vi "04Foot_DAQRead.vi"(0 "task/channels in":refnum<k21>, 7 "number of samples per channel":i32=-1, 9 "timeout":dbl=10.0 format="%0.2f", 11 "error in":errorcluster) -> (4 "task out":refnum<k21>, 6 "data":u8[](array[numeric]), 15 "error out":errorcluster)   [LabVIEW 2015]
doc: "Reads one or more 8-bit unsigned integer samples from a task that contains a single digital input channel. Use an instance that reads 8-bit unsigned integers for devices with up to eight lines per port."
uses:
  nilvaiu.dll
panel:
  in  "depth":i32
  # "sample #"
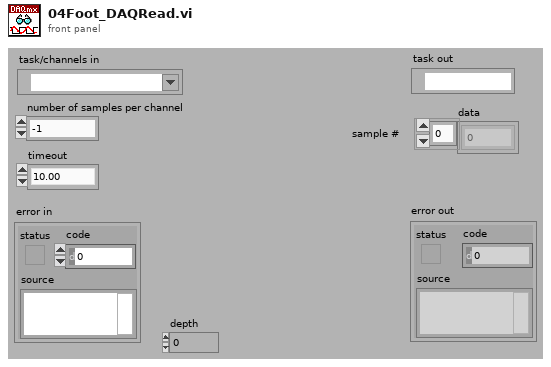
[diagram p1: front panel]
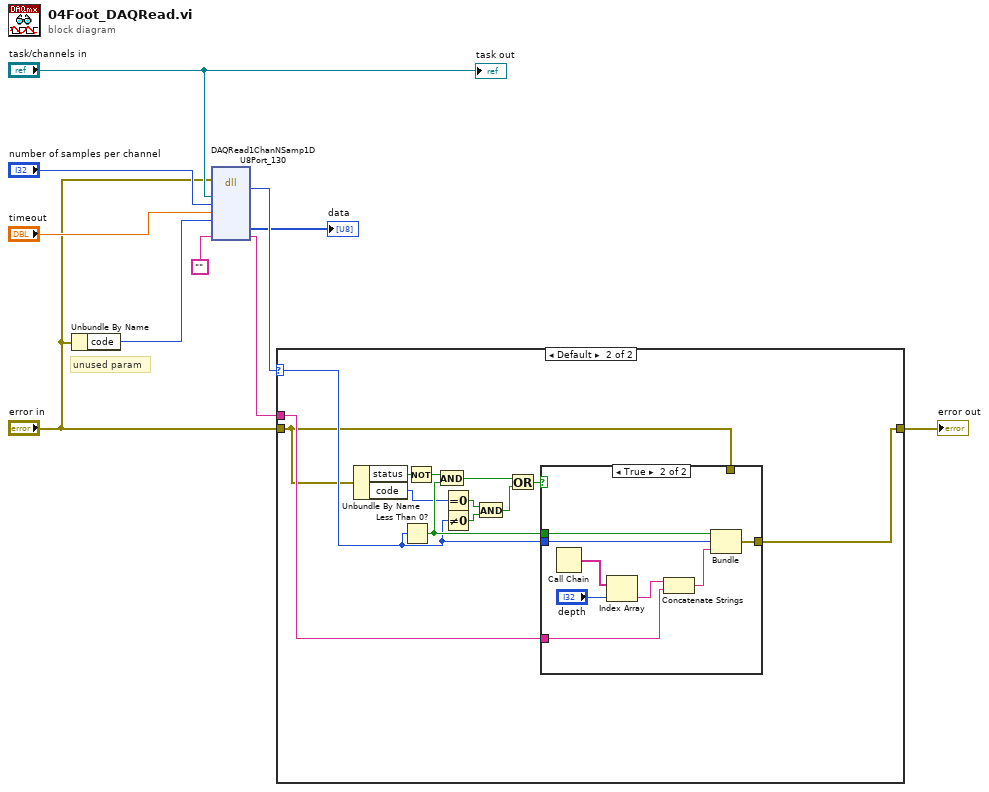
[diagram p0: block diagram]
diagram:
  # "unused param"
  n1 = Unbundle By Name("error in") -> ("code"=w3:i32)
  n2 = dll-call lib="nilvaiu.*" fn="DAQRead1ChanNSamp1DU8Port_130"(error in="error in", "taskID"="task/channels in", "samplesPerChannel"="number of samples per channel", "timeout"="timeout", "incomingStatus"=w3, "extendedErrorInfo"="") -> (w8:i32, "data"=→"data":u8[], "extendedErrorInfo"=w4:string)  [unwired: 6 in, 3 out]
  n3 = case shown="Default" w8 {
    selector: w8 -> [_ w15]
    tunnel: "error in" -> [w11 w12]
    tunnel: [w11 w13] -> w10
    tunnel: w4 -> [_ w14]
    frame 0 {
    }
    frame Default {
      n4 = Unbundle By Name(w12) -> ("status"=w19:bool, "code"=w23:i32)
      n5 = Less Than 0?(x=w15) -> (x < 0?=w24:bool)
      n6 = Not(x=w19) -> (.not. x?=w22:bool)
      n7 = And(x=w22, y=w24) -> (x .and. y?=w20:bool)
      n8 = Equal To 0?(x=w23) -> (x = 0?=w18:bool)
      n9 = Not Equal To 0?(x=w15) -> (x != 0?=w21:bool)
      n10 = And(x=w18, y=w21) -> (x .and. y?=w17:bool)
      n11 = Or(x=w20, y=w17) -> (x .or. y?=w16:bool)
      n12 = case shown="True" w16 {
        tunnel: [w25 w32] -> w13
        tunnel: w15 -> [_ w31]
        tunnel: w24 -> [_ w30]
        tunnel: w12 -> [w25 _]
        tunnel: w14 -> [_ w26]
        frame False {
        }
        frame True {
          n13 = Call Chain() -> (call chain=w29:string[])
          n14 = Index Array(array=w29, index="depth") -> (element=w27:string)
          n15 = Concatenate Strings(w27, w26) -> (w33:string)
          n16 = Bundle(w30, w31, w33) -> (w32:errorcluster)  [unwired: 1 out]
        }
      }
    }
  }
  "error out" <- w10
  "task out" <- "task/channels in"
